vi "Read Configuration Parameters.vi"(8 "error in (no error)":errorcluster, 10 "refnum":T1, 11 "Example Configuration Dialog in":refnum<class "Motor Configuration.lvclass">) -> (0 "error out":errorcluster, 2 "refnum out":T1, 3 "Example Configuration Dialog out":refnum<class "Motor Configuration.lvclass">)   [LabVIEW 2016, in "Hardware.lvlib" / "Motor.lvlib" / "Motor Configuration.lvclass"]
uses:
  <userlib>/Common Components/Hardware/Motor/Motor Config/Motor Configuration.lvclass
  <vilib>/Utility/config.llb/Config Data RefNum.ctl
  <userlib>/Common Components/Hardware/Abstract Hardware/Hardware.lvclass/Hardware.ctl
  <userlib>/Common Components/Hardware/Motor/Motor/Motor.lvclass/Motor.ctl
  <userlib>/Common Components/Hardware/Abstract Hardware/Read Label.vi
  <userlib>/Common Components/Hardware/Abstract Hardware/Read DevInfo.vi
  <userlib>/Common Components/Hardware/Motor/Motor/Motor.lvclass
  C:/Program Files (x86)/National Instruments/LabVIEW 2016/user.lib/Common Components/Hardware/Abstract Hardware/Hardware.lvclass
  <userlib>/Common Components/Hardware/Motor/Motor Config/Accessors/Read Motor Obj.vi
  <userlib>/Common Components/Hardware/Motor/Motor Config/Accessors/Write Motor Obj.vi
  <userlib>/Common Components/Hardware/DevInfo/DevInfo.lvclass
  <vilib>/Utility/config.llb/NI_LVConfig.lvlib
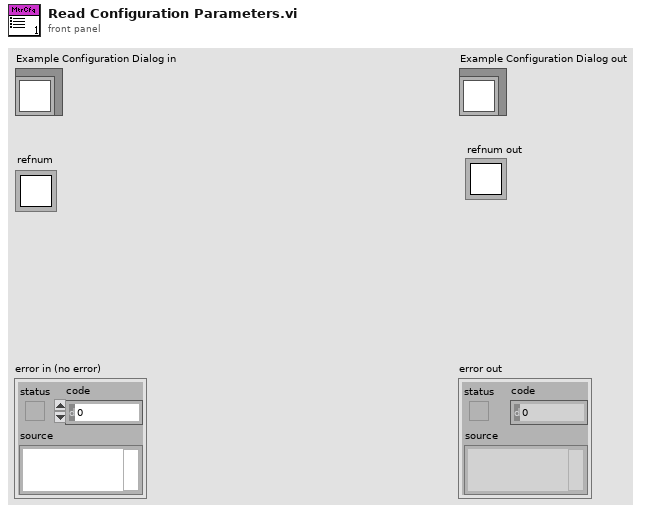
[diagram p1: front panel]
types:
  T1 = typedef "NI_LVConfig.lvlib/Config Data RefNum.ctl" = refnum<k1>
  T2 = typedef "Hardware.lvlib/Motor.lvlib/Motor.lvclass/Motor_Parameters.ctl" = cluster{"closed loop?":bool, "encoder?":bool, "min speed":dbl, "max speed":dbl, "acc time (s)":dbl, "dec time (s)":dbl, "unit mode":enum16{"motor pulses", "real world"}, "motor pulses per revolution":dbl, "display units per motor rev":dbl, "encoder units ratio":dbl, "display unit":string, "display precision":u8, "soft limit min":dbl, "soft limit max":dbl, "Max No. of pull-ins":u8, "Limit+":bool, "Limit+ Logic":enum16{"Low", "High"}, "Limit+ Mode":enum16{"Stop immediately", "Decelerate to Stop"}, "Limit-":bool, "Limit- Logic":enum16{"Low", "High"}, "Limit- Mode":enum16{"Stop immediately", "Decelerate to Stop"}, "Limit+ Sensor ID":enum16{"N/A", "S1", "S2", "S3"}, "Limit- Sensor ID":enum16{"N/A", "S1", "S2", "S3"}, "backlash Compensation":dbl, "soft offset":dbl, "backlash option":enum16{"None", "arriving in + direction", "arriving in - direction"}, "encoder type":enum16{"Linear", "Rotary"}}
  T3 = typedef "Hardware.lvlib/Motor.lvlib/Motor.lvclass/Home Params.ctl" = cluster{"Home Mode":T4, "Home Dir":T5, "Home Pos Shift":dbl}
  T4 = typedef "Hardware.lvlib/Motor.lvlib/Motor.lvclass/Home Mode.ctl" = enum16{"EZ+EL", "EZ only"}
  T5 = typedef "Hardware.lvlib/Motor.lvlib/Motor.lvclass/Home Dir.ctl" = enum16{"negative-", "positive+"}
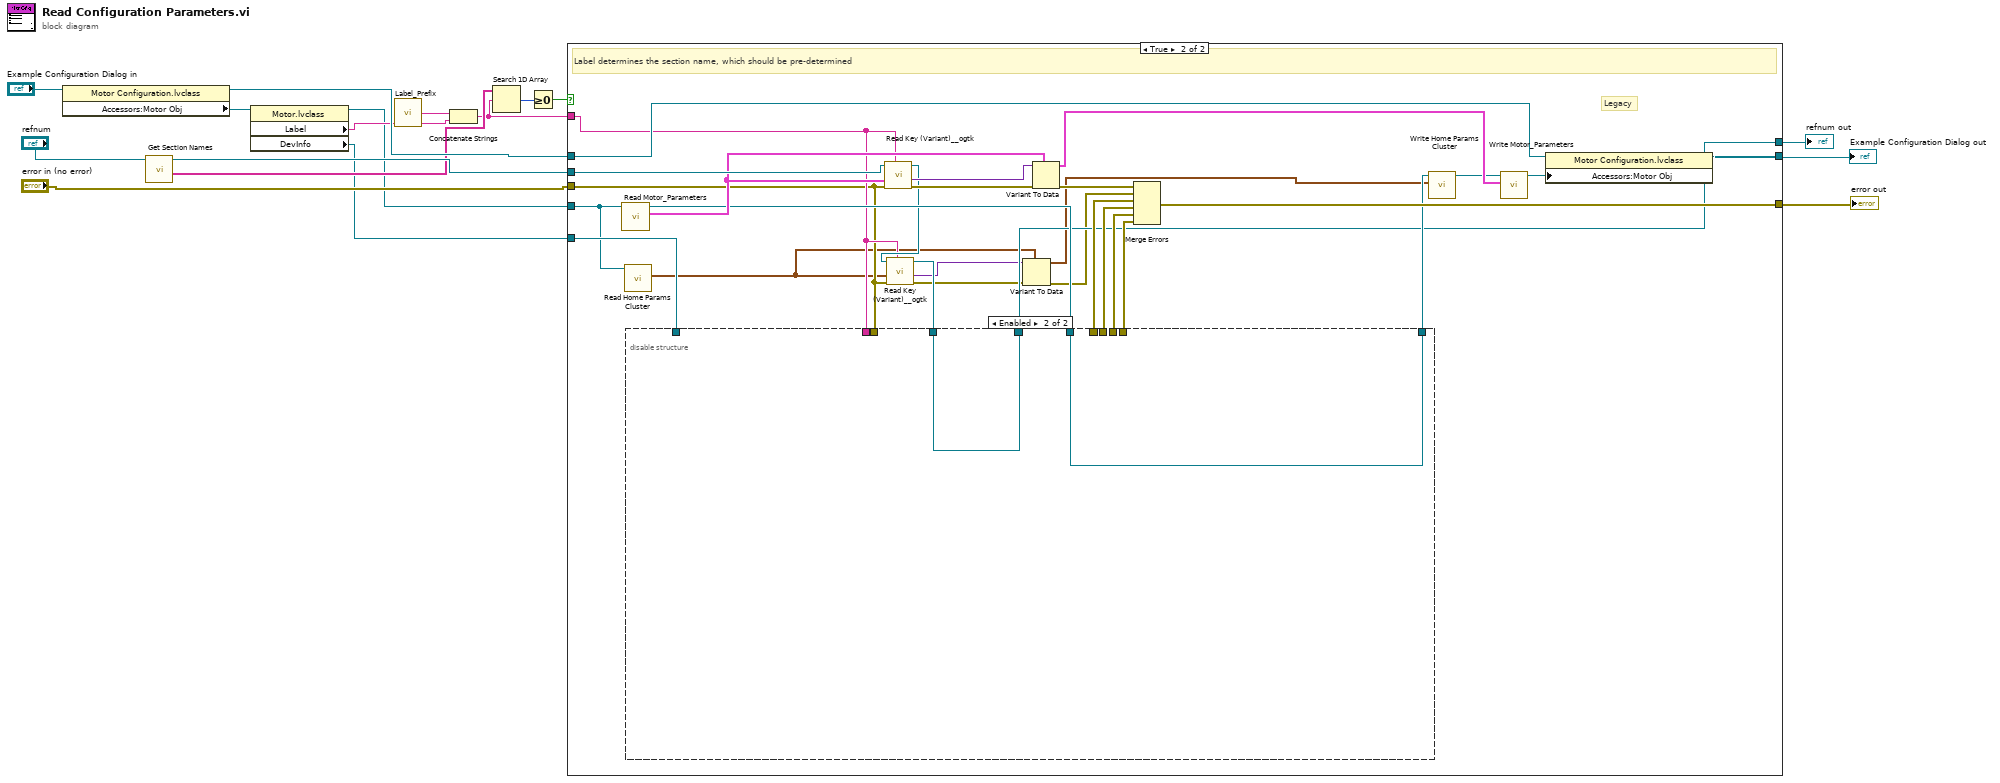
[diagram p0: block diagram]
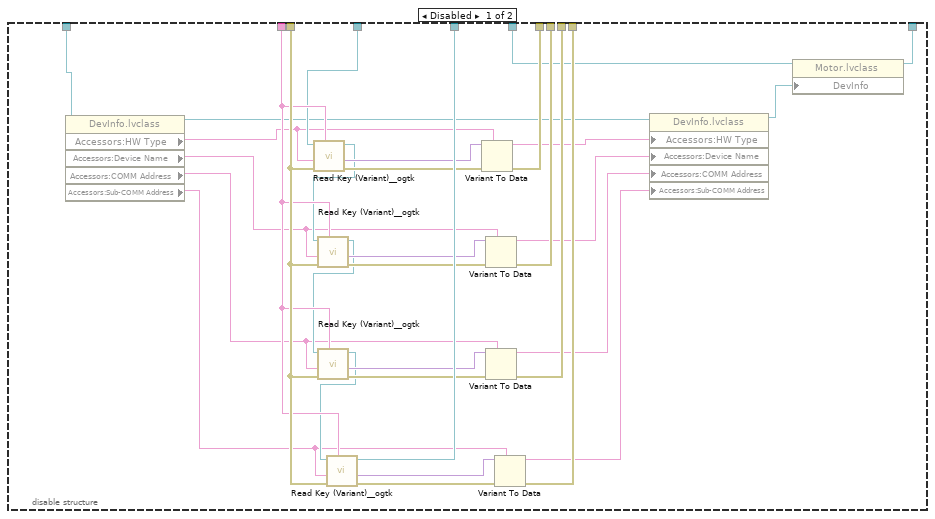
[diagram p3: hidden frame]
diagram:
  n1 = property class="Motor Configuration.lvclass"(reference="Example Configuration Dialog in") -> (reference out=w11:refnum<class "Motor Configuration.lvclass">, "Accessors:Motor Obj"=w9:refnum<class "Motor.lvclass">)  [unwired: 1 in, 1 out]
  n2 = call <vilib>:"Get Section Names.vi"("refnum"="refnum") -> ("section names"=w7:string[], "refnum out"=w8:T1)  [unwired: 8 in, 1 out]
  n3 = property class="Motor.lvclass"(reference=w9) -> (reference out=w2:refnum<class "Motor.lvclass">, "Label"=w3:string, "DevInfo"=w1:refnum<class "DevInfo.lvclass">)  [unwired: 1 in, 1 out]
  n4 = call <userlib>:"Label_Prefix.vi"() -> ("Label Prefix String"=w10:string)
  n5 = Concatenate Strings(w10, w3) -> (w6:string)
  n6 = Search 1D Array(1D array=w7, element=w6) -> (index of element=w5:i32)  [unwired: 1 in]
  n7 = Greater Or Equal To 0?(x=w5) -> (x >= 0?=w4:bool)
  n8 = case shown="True" w4 {
    tunnel: w8 -> [w19 w49]
    tunnel: "error in (no error)" -> [w18 w28]
    tunnel: w11 -> [w20 w34]
    tunnel: [w20 w35] -> w15
    tunnel: [w19 w33] -> w14
    tunnel: [w18 w48] -> w13
    tunnel: w6 -> [_ w29]
    tunnel: w2 -> [_ w32]
    tunnel: w1 -> [_ w39]
    frame False {
    }
    frame True {
      # "Legacy"
      # "Label determines the section name, which should be pre-determined"
      n9 = call <userlib>:"Read Motor_Parameters.vi"("Motor in"=w32) -> ("motor parameters"=w40:T2, "Motor out"=w38:refnum<class "Motor.lvclass">)  [unwired: 8 in, 1 out]
      n10 = call <userlib>:"Read Home Params Cluster.vi"("Motor in"=w32) -> ("Home Params Cluster"=w25:T3)  [unwired: 8 in, 2 out]
      n11 = call <userlib>:"Read Key (Variant)__ogtk.vi"("section"=w29, "error in (no error)"=w28, "type"=w40, "refnum"=w49) -> ("error out"=w46:errorcluster, "key-value"=w47:variant, "refnum out"=w31:T1)  [unwired: 4 in, 1 out]
      n12 = call <userlib>:"Read Key (Variant)__ogtk.vi"("section"=w29, "error in (no error)"=w28, "type"=w25, "refnum"=w31) -> ("error out"=w27:errorcluster, "key-value"=w26:variant, "refnum out"=w30:T1)  [unwired: 4 in, 1 out]
      n13 = disable-structure shown="Enabled" {
        disable-tunnel: w28 -> [w81 _]
        disable-tunnel: w29 -> [w80 _]
        disable-tunnel: [w79 w82] -> w33
        disable-tunnel: [w67 _] -> w44
        disable-tunnel: [w66 _] -> w43
        disable-tunnel: [w65 _] -> w42
        disable-tunnel: [w64 _] -> w41
        disable-tunnel: w30 -> [w63 w82]
        disable-tunnel: w39 -> [w62 _]
        disable-tunnel: w38 -> [w57 w83]
        disable-tunnel: [w51 w83] -> w36
        frame Disabled {
          n14 = property class="DevInfo.lvclass"(reference=w62) -> (reference out=w56:refnum<class "DevInfo.lvclass">, "Accessors:HW Type"=w61:string, "Accessors:Device Name"=w60:string, "Accessors:COMM Address"=w59:string, "Accessors:Sub-COMM Address"=w58:string)  [unwired: 1 in, 1 out]
          n15 = call <userlib>:"Read Key (Variant)__ogtk.vi"("section"=w80, "error in (no error)"=w81, "type"=w61, "refnum"=w63) -> ("error out"=w77:errorcluster, "key-value"=w78:variant, "refnum out"=w70:T1)  [unwired: 4 in, 1 out]
          n16 = call <userlib>:"Read Key (Variant)__ogtk.vi"("section"=w80, "error in (no error)"=w81, "type"=w60, "refnum"=w70) -> ("error out"=w75:errorcluster, "key-value"=w76:variant, "refnum out"=w69:T1)  [unwired: 4 in, 1 out]
          n17 = call <userlib>:"Read Key (Variant)__ogtk.vi"("section"=w80, "error in (no error)"=w81, "type"=w59, "refnum"=w69) -> ("error out"=w73:errorcluster, "key-value"=w74:variant, "refnum out"=w68:T1)  [unwired: 4 in, 1 out]
          n18 = call <userlib>:"Read Key (Variant)__ogtk.vi"("section"=w80, "error in (no error)"=w81, "type"=w58, "refnum"=w68) -> ("error out"=w71:errorcluster, "key-value"=w72:variant, "refnum out"=w79:T1)  [unwired: 4 in, 1 out]
          n19 = Variant To Data(error in=w77, type=w61, Variant=w78) -> (data=w55:string, error out=w67:errorcluster)
          n20 = Variant To Data(error in=w75, type=w60, Variant=w76) -> (data=w54:string, error out=w66:errorcluster)
          n21 = Variant To Data(error in=w73, type=w59, Variant=w74) -> (data=w53:string, error out=w65:errorcluster)
          n22 = Variant To Data(error in=w71, type=w58, Variant=w72) -> (data=w52:string, error out=w64:errorcluster)
          n23 = property class="DevInfo.lvclass"(reference=w56, "Accessors:HW Type"=w55, "Accessors:Device Name"=w54, "Accessors:COMM Address"=w53, "Accessors:Sub-COMM Address"=w52) -> (reference out=w50:refnum<class "DevInfo.lvclass">)  [unwired: 1 in, 1 out]
          n24 = property class="Motor.lvclass"(reference=w57, "DevInfo"=w50) -> (reference out=w51:refnum<class "Motor.lvclass">)  [unwired: 1 in, 1 out]
        }
        frame Enabled {
        }
      }
      n25 = Variant To Data(error in=w27, type=w25, Variant=w26) -> (data=w22:T3, error out=w23:errorcluster)
      n26 = Variant To Data(error in=w46, type=w40, Variant=w47) -> (data=w37:T2, error out=w45:errorcluster)
      n27 = Merge Errors(w45, w23, w44, w43, w42, w41) -> (w48:errorcluster)
      n28 = call <userlib>:"Write Home Params Cluster.vi"("Home Params Cluster"=w22, "Motor in"=w36) -> ("Motor out"=w24:refnum<class "Motor.lvclass">)  [unwired: 8 in, 1 out]
      n29 = call <userlib>:"Write Motor_Parameters.vi"("motor parameters"=w37, "Motor in"=w24) -> ("Motor out"=w21:refnum<class "Motor.lvclass">)  [unwired: 8 in, 1 out]
      n30 = property class="Motor Configuration.lvclass"(reference=w34, "Accessors:Motor Obj"=w21) -> (reference out=w35:refnum<class "Motor Configuration.lvclass">)  [unwired: 1 in, 1 out]
    }
  }
  "Example Configuration Dialog out" <- w15
  "error out" <- w13
  "refnum out" <- w14
